vi "ConnectionTest.vi"() -> ()   [LabVIEW 2015]
panel:
  in  "Stop Button":bool
  out "Response":string
  out "CommandSended":bool
  in  "Command":string="WX,PRG=0000,BLK=000,CharacterString=\"HelloWord\""
  in  "SendComand":bool
  in  "listening port":u16=50002
  in  "Laser IP address":string="192.168.0.11"
  # "TCP"
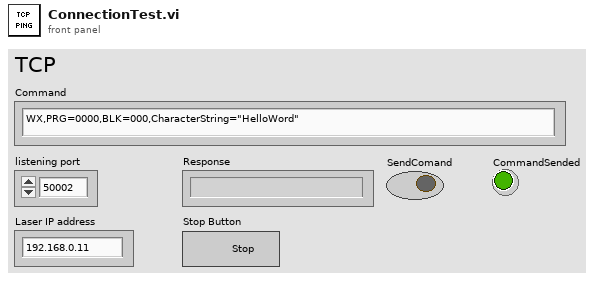
[diagram p1: front panel]
types:
  T1 = enum16{"Standard", "Buffered", "CRLF", "Immediate"}
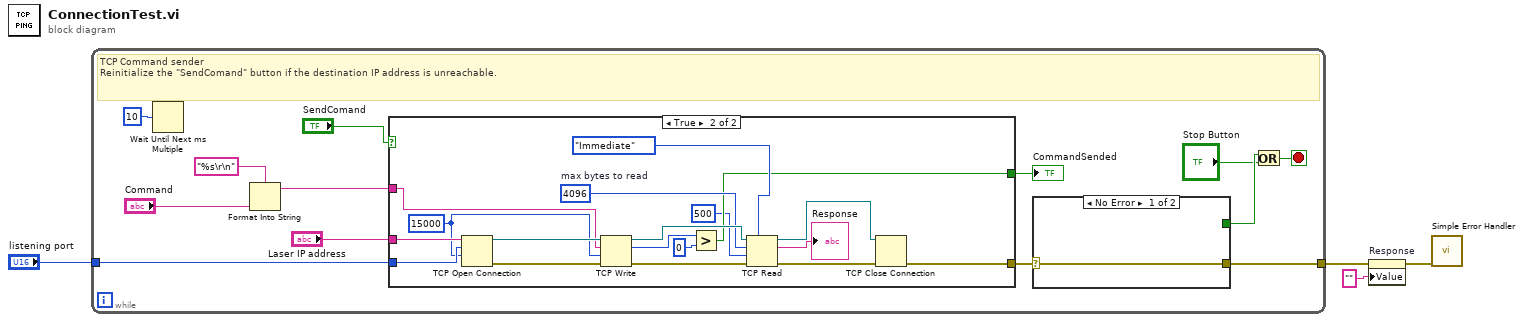
[diagram p0: block diagram]
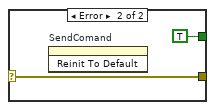
[diagram p2: hidden frame]
diagram:
  n1 = while {
    tunnel: "listening port" -> [w9]
    tunnel: [w8] -> w3
    stop <- w5 stop-if-true
    # "TCP Command sender\nReinitialize the \"SendComand\" button if the destination IP address is unreachable."
    n2 = Wait Until Next ms Multiple(millisecond multiple=u32 10) -> ()  [unwired: 1 out]
    n3 = Format Into String "Format Into String"(format string="%s\r\n", "Command") -> (resulting string=w14:string)  [unwired: 2 in, 1 out]
    n4 = case shown="True" "SendComand" {
      tunnel: [_ w28] -> w12
      tunnel: w14 -> [_ w27]
      tunnel: "Laser IP address" -> [_ w38]
      tunnel: w9 -> [_ w37]
      tunnel: [_ w25] -> w10
      frame False {
      }
      frame True {
        w31 = 4096  # max bytes to read
        w34 = 15000 ("timeout ms (60000)")
        n5 = TCP Open Connection(address=w38, remote port or service name=w37, timeout ms (60000)=w34) -> (connection ID=w35:refnum<k5>, error out=w36:errorcluster)  [unwired: 2 in]
        n6 = TCP Write(connection ID=w35, data in=w27, error in (no error)=w36, 9:w34) -> (connection ID out=w33:refnum<k5>, bytes written=w22:i32, error out=w32:errorcluster)
        n7 = Greater?(x=w22, y=0) -> (0:w25:bool)
        n8 = TCP Read(connection ID=w33, bytes to read=w31, error in (no error)=w32, 7:T1."Immediate" ("mode (standard)"), 9:500 ("timeout ms (25000)")) -> (connection ID out=w29:refnum<k5>, data out=→"Response":string, error out=w30:errorcluster)
        n9 = TCP Close Connection(connection ID=w29, error in (no error)=w30) -> (error out=w28:errorcluster)  [unwired: 1 in, 1 out]
      }
    }
    "CommandSended" <- w10
    n10 = case shown="No Error" w12 {
      selector: w12 -> [w18 w19]
      tunnel: [_ TRUE] -> w7
      tunnel: [w18 w19] -> w8
      frame No Error {
      }
      frame Error {
        n11 = invoke on="SendComand" class="Bool" method="Reinit To Default"() -> ()  [unwired: 3 in, 3 out]
      }
    }
    n12 = Or(x=w7, y="Stop Button") -> (x .or. y?=w5:bool)
  }
  n13 = property on="Response" class="Str"(error in=w3, "Value"="" ("data out")) -> (error out=w2:errorcluster)  [unwired: 1 in, 1 out]
  n14 = call <vilib>:"Simple Error Handler.vi"("error in (no error)"=w2) -> ()  [unwired: 4 in, 5 out]
